vi "AC_withrepeatStates_Test.vi"() -> ()   [LabVIEW 2017]
panel:
  out "Iterations":i32
  out "Pass":bool
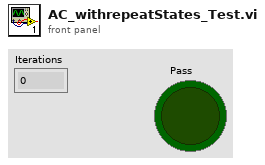
[diagram p1: front panel]
types:
  T1 = enum16{"open", "replace", "create", "open or create", "replace or create", "replace or create with confirmation"}
  T2 = cluster{"[0]":string, "[1]":string, "[2]":string, "[3]":string, "[4]":string, "[5]":string, "[6]":string, "[7]":string, "[8]":string}
  T3 = cluster{"call chain[0]":string, "call chain[1]":string, "call chain[2]":string, "call chain[3]":string, "call chain[4]":string, "call chain[5]":string, "call chain[6]":string, "call chain[7]":string, "call chain[8]":string}
  T4 = cluster{"ENIPath":path, "Iterations":i32, "DelayBetweenIterations":i32, "TimeStamp":string, "TestSuite":string, "ReportPath":path}
  T5 = cluster{"SPI_BaudRate":u32, "EtherCAT_Static_IP":string, "SPI_Parity":u16, "SPI_DataBits":u16, "SPI_StopBits":u16, "SPI_FlowControl":u16, "Global_ReportPath":path, "AC_ENIPath":path, "PC_ENIPath":path}
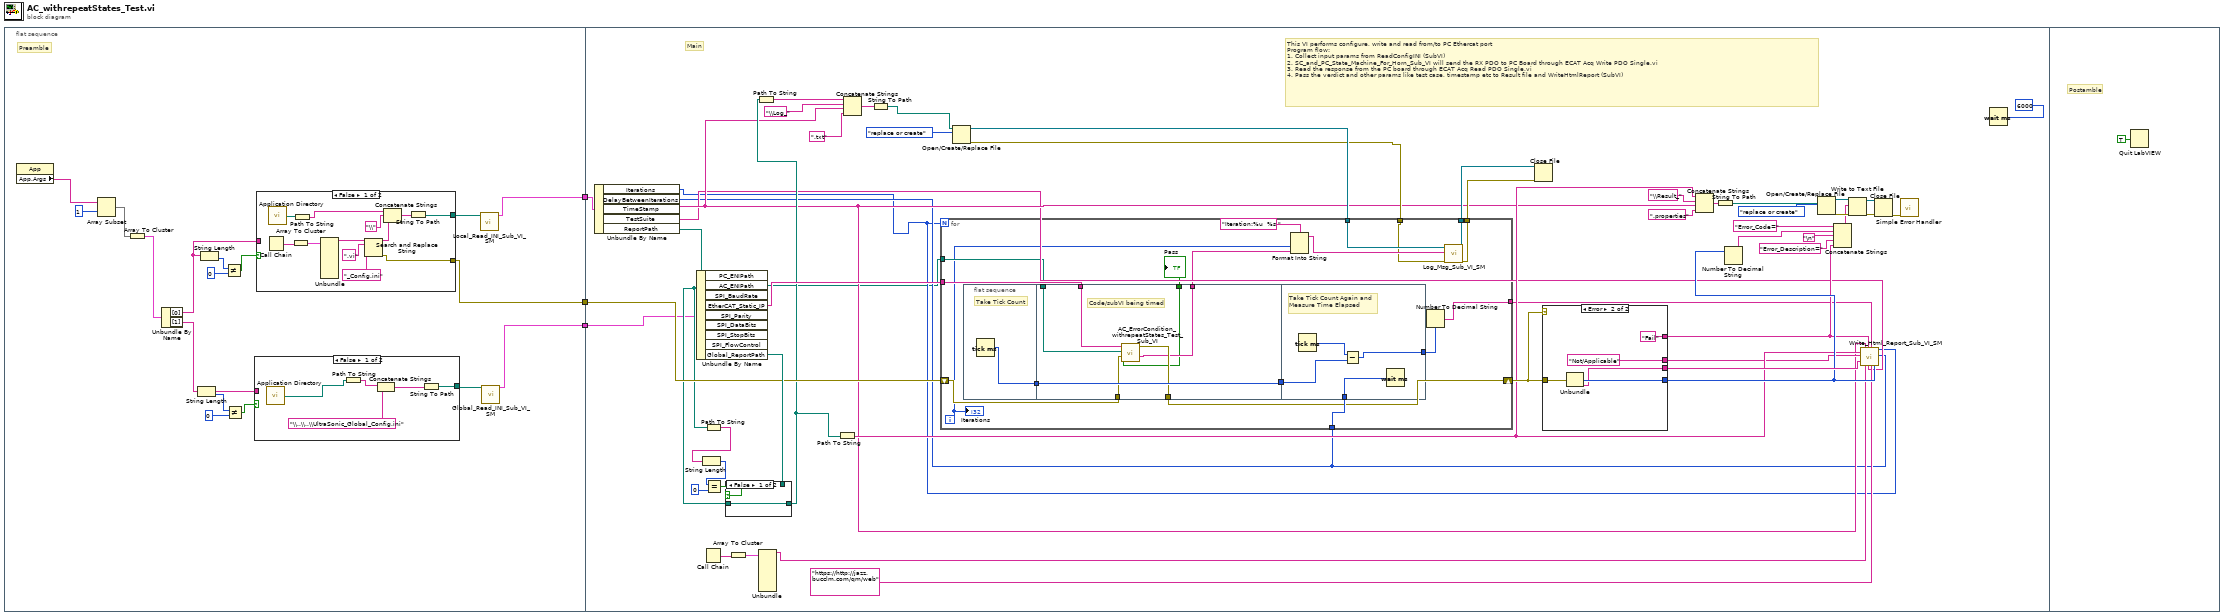
[diagram p0: block diagram]
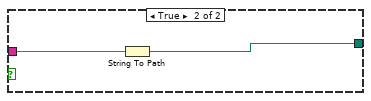
[diagram p2: hidden frame]
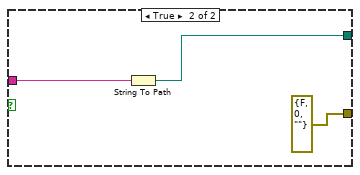
[diagram p3: hidden frame]
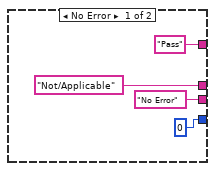
[diagram p5: hidden frame]
diagram:
  n1 = flat-sequence {
    tunnel: [w6] -> w3
    tunnel: [w5] -> w2
    tunnel: [w4] -> w1
    tunnel: w3 -> [w68]
    tunnel: w2 -> [w50]
    tunnel: w1 -> [w44]
    frame #0 {
      # "Preamble"
      n2 = property class="App"() -> ("App.Args"=w8:string[])  [unwired: 2 in, 2 out]
      n3 = Array Subset(array=w8, index=1) -> (w9:string[])  [unwired: 1 in]
      n4 = Array To Cluster(array=w9) -> (cluster=w10:T2)
      n5 = Unbundle By Name(w10) -> ("[0]"=w14:string, "[1]"=w17:string)
      n6 = String Length(string=w17) -> (length=w18:i32)
      n7 = String Length(string=w14) -> (length=w11:i32)
      n8 = Not Equal?(x=w11, y=0) -> (x != y?=w13:bool)
      n9 = Not Equal?(x=w18, y=0) -> (x != y?=w16:bool)
      n10 = case shown="False" w16 {
        tunnel: [w22 w27] -> w20
        tunnel: w17 -> [_ w26]
        frame False {
          n11 = call <vilib>:"Application Directory.vi"() -> ("Application Directory"=w21:path)
          n12 = Path To String(path=w21) -> (string=w25:string)
          n13 = Concatenate Strings(w25, "\\..\\..\\UltraSonic_Global_Config.ini" ("string")) -> (w23:string)
          n14 = String To Path(string=w23) -> (path=w22:path)
        }
        frame True {
          n15 = String To Path(string=w26) -> (path=w27:path)
        }
      }
      n16 = case shown="False" w13 {
        tunnel: w14 -> [_ w42]
        tunnel: [w39 w41] -> w19
        tunnel: [w28 errorcluster {"status"=FALSE, "code"=0, "source"=""} ("error out")] -> w6
        frame False {
          n17 = Call Chain() -> (call chain=w37:string[])
          n18 = call <vilib>:"Application Directory.vi"() -> ("Application Directory"=w38:path)
          n19 = Array To Cluster(array=w37) -> (cluster=w36:T3)
          n20 = Path To String(path=w38) -> (string=w30:string)
          n21 = Unbundle(w36) -> ("call chain[0]"=w35:string)  [unwired: 8 out]
          n22 = Search and Replace String(input string=w35, search string=".vi", replace string="_Config.ini" ("replace string (\"\")")) -> (result string=w32:string, error out=w28:errorcluster)  [unwired: 5 in, 2 out]
          n23 = Concatenate Strings(w30, "\\" ("string"), w32) -> (w29:string)
          n24 = String To Path(string=w29) -> (path=w39:path)
        }
        frame True {
          n25 = String To Path(string=w42) -> (path=w41:path)
        }
      }
      n26 = call "Local_Read_INI_Sub_VI_SM.vi"("Config File Path"=w19) -> ("output cluster"=w5:T4)  [unwired: 10 in]
      n27 = call "Global_Read_INI_Sub_VI_SM.vi"("Config File Path"=w20) -> ("output cluster"=w4:T5)  [unwired: 14 in]
    }
    frame #1 {
      # "This VI performs configure, write and read from/to PC Ethercat port\nProgram flow:\n1. Collect input params from ReadConfigINI (SubVI)\n2. SC_and_PC_State_Machine_For_Horn_Sub_VI will send the RX PDO to PC Board through ECAT Acq Write PDO Single.vi \n3. Read the response from the PC board through ECAT Acq Read PDO Single.vi \n4. Pass the verdict and other params like test case, timestamp etc to Result file and WriteHtmlReport (SubVI)"
      # "Main"
      n28 = Unbundle By Name(w50) -> ("Iterations"=w45:i32, "DelayBetweenIterations"=w46:i32, "TimeStamp"=w48:string, "TestSuite"=w47:string, "ReportPath"=w49:path)
      n29 = Unbundle By Name(w44) -> ("AC_ENIPath"=w43:path, "EtherCAT_Static_IP"=w70:string, "Global_ReportPath"=w88:path)  [unwired: 6 out]
      n30 = Path To String(path=w49) -> (string=w92:string)
      n31 = String Length(string=w92) -> (length=w91:i32)
      n32 = Call Chain() -> (call chain=w94:string[])
      n33 = Equal?(x=w91, y=0) -> (x = y?=w89:bool)
      n34 = case shown="False" w89 {
        tunnel: w88 -> [_ w127]
        tunnel: [w126 w127] -> w55
        tunnel: w49 -> [w126 _]
        frame False {
        }
        frame True {
        }
      }
      n35 = Array To Cluster(array=w94) -> (cluster=w93:T3)
      n36 = Path To String(path=w55) -> (string=w58:string)
      n37 = Unbundle(w93) -> ("call chain[0]"=w63:string)  [unwired: 8 out]
      n38 = Path To String(path=w55) -> (string=w65:string)
      n39 = Concatenate Strings(w58, "\\Log_" ("string"), w48, ".txt" ("string")) -> (w60:string)
      n40 = String To Path(string=w60) -> (path=w59:path)
      n41 = Open/Create/Replace File(file path (use dialog)=w59, operation (0:open)=T1."replace or create") -> (refnum out=w54:refnum<file>, error out=w51:errorcluster)  [unwired: 1 in, 4 out]
      n42 = for {
        N: w45 -> [_]
        tunnel: w70 -> [w111]
        tunnel: w43 -> [w110]
        tunnel: [w108] -> w64
        shift-right: [w97] -> w67
        shift-left: w68 -> [w109]
        tunnel: w54 -> [w106]
        tunnel: [w105] -> w53
        tunnel: [w104] -> w52
        tunnel: w51 -> [w99]
        tunnel: w46 -> [w98]
        i -> [w103]
        n43 = flat-sequence {
          tunnel: [w114] -> w113
          tunnel: [w121] -> w112
          tunnel: w113 -> [w121]
          tunnel: w111 -> [w119]
          tunnel: w110 -> [w118]
          tunnel: w109 -> [w117]
          tunnel: [w115] -> w107
          tunnel: [w120] -> w97
          tunnel: [w116] -> w96
          tunnel: w112 -> [w125]
          tunnel: [w123] -> w102
          tunnel: w98 -> [w122]
          frame #0 {
            # "Take Tick Count"
            n44 = Tick Count (ms)() -> (millisecond timer value=w114:u32)
          }
          frame #1 {
            # "Code/subVI being timed"
            n45 = call "AC_ErrorCondition_withrepeatStates_Test_Sub_VI.vi"("error in"=w117, "Path ENI File"=w118, "IP NIC"=w119) -> ("Data values from SC and AC"=w116:string, "error out"=w120:errorcluster, "Pass"=w115:bool)  [unwired: 6 in]
          }
          frame #2 {
            # "Take Tick Count Again and Measure Time Elapsed"
            n46 = Tick Count (ms)() -> (millisecond timer value=w124:u32)
            n47 = Subtract(x=w124, y=w125) -> (x-y=w123:u32)
            n48 = Wait (ms)(milliseconds to wait=w122) -> ()  [unwired: 1 out]
          }
        }
        n49 = Format Into String(format string="Iteration:%u  %s ", w103, w96) -> (resulting string=w100:string)  [unwired: 2 in, 1 out]
        n50 = Number To Decimal String(number=w102) -> (decimal integer string=w108:string)  [unwired: 1 in]
        n51 = call "Log_Msg_Sub_VI_SM.vi"("error in (no error)"=w99, "String"=w100, "Byte Stream File in"=w106) -> ("error out"=w105:errorcluster, "Byte Stream File out"=w104:refnum<file>)  [unwired: 7 in]
        "Pass" <- w107
        "Iterations" <- w103
      }
      n52 = Close File(refnum=w52, error in=w53) -> ()  [unwired: 2 out]
      n53 = case shown="Error" w67 {
        tunnel: ["Pass" "Fail"] -> w71
        tunnel: w67 -> [_ w135]
        tunnel: [0 ("code") w134] -> w75
        tunnel: ["No Error" ("source") w133] -> w95
        tunnel: ["Not/Applicable" "Not/Applicable"] -> w62
        frame No Error {
        }
        frame Error {
          n54 = Unbundle(w135) -> ("code"=w134:i32, "source"=w133:string)  [unwired: 1 out]
        }
      }
      n55 = Concatenate Strings(w65, "\\Result_" ("string"), w48, ".properties" ("string")) -> (w87:string)
      n56 = String To Path(string=w87) -> (path=w79:path)
      n57 = Number To Decimal String(number=w75) -> (decimal integer string=w74:string)  [unwired: 1 in]
      n58 = Open/Create/Replace File(file path (use dialog)=w79, operation (0:open)=T1."replace or create") -> (refnum out=w78:refnum<file>, error out=w83:errorcluster)  [unwired: 4 in, 1 out]
      n59 = Concatenate Strings("Error_Code=" ("string"), w74, "\n", "Error_Description=" ("string"), w71) -> (w77:string)
      n60 = Write to Text File(file (use dialog)=w78, text=w77, error in=w83) -> (refnum out=w82:refnum<file>, error out=w81:errorcluster)  [unwired: 1 in, 1 out]
      n61 = call "Write_Html_Report_Sub_VI_SM.vi"("ReprtPath"=w65, "Remarks"=w62, "Error Description"=w95, "Timestamp"=w48, "TestCase"=w63, "Verdict"=w71, "TestSuite"=w47, "Time taken to execute  test in msec"=w64, "JazzDashboardLink"="https://http://jazz.bucclm.com/qm/web" ("TestSuite"), "Error Code"=w75, "Number of times test executed (Iterations)"=w45, "Delay Between Iterations"=w46) -> ()  [unwired: 8 in]
      n62 = Close File(refnum=w82, error in=w81) -> (error out=w80:errorcluster)  [unwired: 1 out]
      n63 = call <vilib>:"Simple Error Handler.vi"("error in (no error)"=w80) -> ()  [unwired: 4 in, 5 out]
      n64 = Wait (ms)(milliseconds to wait=u32 6000) -> ()  [unwired: 1 out]
    }
    frame #2 {
      # "Postamble"
      n65 = Quit LabVIEW(quit? (T)=TRUE) -> ()
    }
  }
